vi "SPI_SET_3W_Mode.vi"   [LabVIEW 2019]
doc: "initialise the chip in 3 wires mode"
uses:
  <vilib>/rvi/eio/common/nirviEmuTemplateMethod_errors.vi
  <vilib>/eio/EIONode/EIONode.xnode
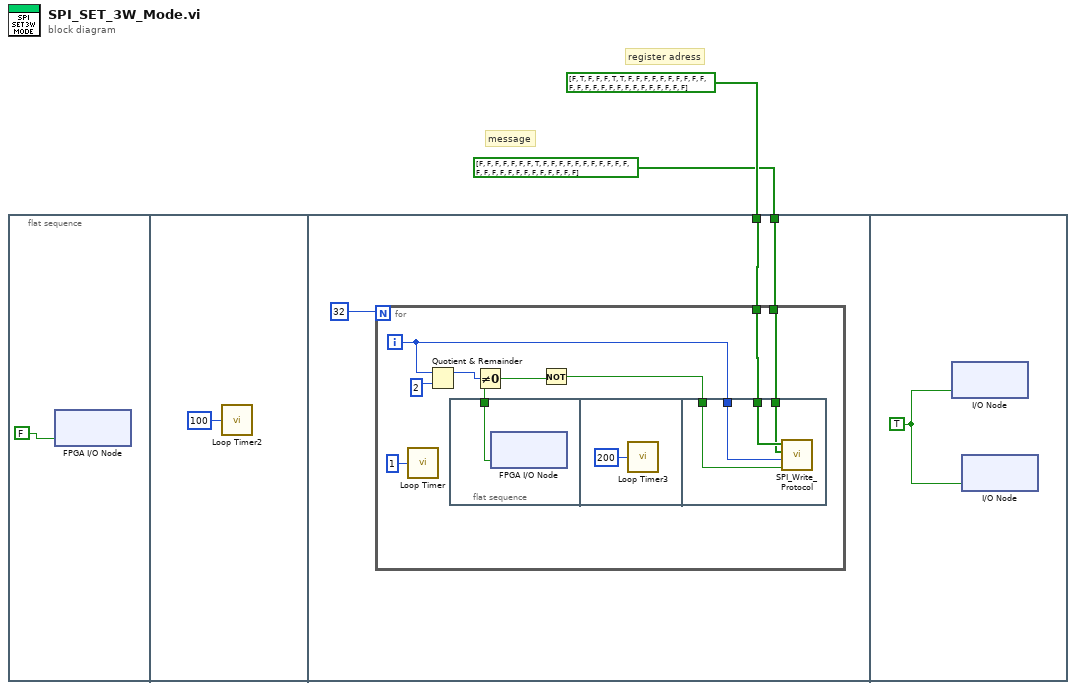
[diagram p0: block diagram]
diagram:
  # "message"
  # "register adress"
  n1 = flat-sequence {
    tunnel: bool[] [FALSE, TRUE, FALSE, FALSE, FALSE, TRUE, TRUE, FALSE, FALSE, FALSE, FALSE, FALSE, FALSE, FALSE, FALSE, FALSE, FALSE, FALSE, FALSE, FALSE, FALSE, FALSE, FALSE, FALSE, FALSE, FALSE, FALSE, FALSE, FALSE, FALSE, FALSE, FALSE] ("Register_adress") -> [w6]
    tunnel: bool[] [FALSE, FALSE, FALSE, FALSE, FALSE, FALSE, FALSE, TRUE, FALSE, FALSE, FALSE, FALSE, FALSE, FALSE, FALSE, FALSE, FALSE, FALSE, FALSE, FALSE, FALSE, FALSE, FALSE, FALSE, FALSE, FALSE, FALSE, FALSE, FALSE, FALSE, FALSE, FALSE] ("message") -> [w5]
    frame #0 {
      n2 = xnode "FPGA I/O Node"("CS"=FALSE) -> ()  [unwired: 1 in, 1 out]
    }
    frame #1 {
      n3 = call "Loop Timer2"("Count(uSec)"=u32 100 ("Count(Ticks)")) -> ()  [unwired: 1 out]
    }
    frame #2 {
      n4 = for {
        N: 32 -> [_]
        tunnel: w6 -> [w11]
        tunnel: w5 -> [w10]
        i -> [w12]
        n5 = call "Loop Timer"("Count(mSec)"=u32 1) -> ()  [unwired: 1 out]
        n6 = Quotient & Remainder(x=w12, y=2) -> (x-y*floor(x/y)=w14:i32)  [unwired: 1 out]
        n7 = flat-sequence {
          tunnel: w9 -> [w16]
          tunnel: w8 -> [w20]
          tunnel: w12 -> [w21]
          tunnel: w11 -> [w19]
          tunnel: w10 -> [w18]
          frame #0 {
            n8 = xnode "FPGA I/O Node"("SCL"=w16) -> ()  [unwired: 1 in, 1 out]
          }
          frame #1 {
            n9 = call "Loop Timer3"("Count(uSec)"=u32 200 ("Count(mSec)")) -> ()  [unwired: 1 out]
          }
          frame #2 {
            n10 = call "SPI_Write_Protocol.vi"("rising_edge"=w20, "bit_index"=w21, "message"=w18, "Register_adress"=w19) -> ()  [unwired: 8 in]
          }
        }
        n11 = Not Equal To 0?(x=w14) -> (x != 0?=w9:bool)
        n12 = Not(x=w9) -> (.not. x?=w8:bool)
      }
    }
    frame #3 {
      w22 = TRUE ("CS")
      n13 = xnode "I/O Node"("CS"=w22) -> ()  [unwired: 1 in, 1 out]
      n14 = xnode "I/O Node"("SCL"=w22) -> ()  [unwired: 1 in, 1 out]
    }
  }
